vi "Launch ExampleDependency.vi"(8 "error in (no error)":errorcluster, 11 "SMO.Example in":refnum<class "SMO.Example.lvclass">) -> (0 "error out":errorcluster, 3 "SMO.Example out":refnum<class "SMO.Example.lvclass">)   [LabVIEW 2013, in "SMO.Example.lvclass"]
uses:
  SMO.Example.lvclass
  SMO/SMO.lvclass
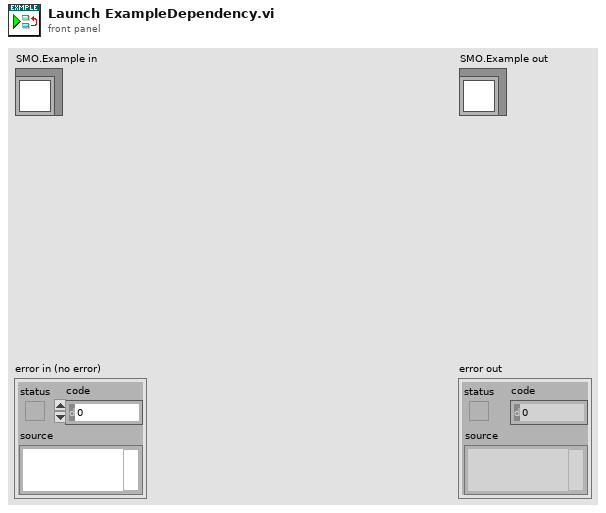
[diagram p1: front panel]
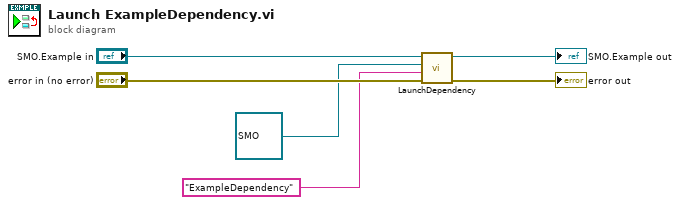
[diagram p0: block diagram]
diagram:
  n1 = call "LaunchDependency.vi"("error in (no error)"="error in (no error)", "Dependency Name"="ExampleDependency", "Dependency Type"=refnum<class "SMO.lvclass"> refnum ("SMO.lvclass"), "SMO in"="SMO.Example in") -> ("error out"=→"error out":errorcluster, "SMO out"=→"SMO.Example out":refnum<class "SMO.Example.lvclass">)  [unwired: 4 in, 2 out]
